vi "Dashboard Main.vi"() -> ()   [LabVIEW 2016]
uses:
  <vilib>/Utility/miscctls.llb/LVRowAndColumnTypeDef.ctl
  <vilib>/event_ctls.llb/eventvkey.ctl
  <vilib>/Rock Robotics/Network Tables/NT Read Numeric Array.vi
  <vilib>/Rock Robotics/WPI/Dashboard/WPI_DashboardLogging Global.vi
  <vilib>/Instr/_visa.llb/VISA Configure Serial Port (Instr).vi
panel:
  in  "Camera Settings Right":T1={"Frame Rate"=30, "Compression"=30, "Size"=1, "DB Camera Config"=FALSE} {"Frame Rate" scale=1.0..30.0; "Compression" scale=100.0..-1.0; "Size" items=["640x480", "320x240", "160x120"]}
  in  "Camera Name Right":string(combo)="No Camera Selection"
  out "Camera Info":cluster{"Mbps LED":bool, "Mbps":dbl, "fps":dbl} {"fps" format="%#.1g"; "Mbps" format="%#.1g"}
  in  "Camera Settings":T1={"Frame Rate"=30, "Compression"=30, "Size"=1, "DB Camera Config"=FALSE} {"Frame Rate" scale=1.0..30.0; "Compression" scale=100.0..-1.0; "Size" items=["640x480", "320x240", "160x120"]}
  in  "TCP":refnum<k5>
  in  "Rec Mode":enum32{"Stop", "Record", "Playback"}(radio)
  out "Robot IP":string
  out "Image Message":string="Timeout in Camera Communications"
  in  "Dashboard Tab":T2(tab)
  out "Boutton":bool
  out "Led2 prevstate":bool
  in  "Led2":bool
  out "Led1 prevstate":bool
  in  "Led1":bool
  in  "Select Auto":string(combo)="Select Autonomous ..."
  out "NT Connection":bool
  out "MotorChart R":cluster{"Numeric":dbl, "Numeric":dbl}(graph)
  out "MotorChart L":cluster{"Numeric":dbl, "Numeric":dbl}(graph)
  out "MotorSliders R":cluster{"MotorSlide1":dbl, "MotorSlide2":dbl} {"MotorSlide2" scale=-1.0..1.0 scale format="%#_2e"; "MotorSlide1" scale=-1.0..1.0 scale format="%#_2e"}
  out "MotorSliders L":cluster{"MotorSlide1":dbl, "MotorSlide2":dbl} {"MotorSlide2" scale=-1.0..1.0 scale format="%#_2e"; "MotorSlide1" scale=-1.0..1.0 scale format="%#_2e"}
  out "Gyro":dbl(knob) scale=0.0..360.0
  out "JS1 Z":dbl(slide) scale=-1.0..1.0 scale format="%#_2e"
  out "JS1 Graph":cluster{"X":dbl, "Y":dbl}[](graph)
  out "JS1 Buttons":T3
  out "JS2 Z":dbl(slide) scale=-1.0..1.0 scale format="%#_2e"
  out "JS2 Graph":cluster{"X":dbl, "Y":dbl}[](graph)
  out "JS2 Buttons":T3
  out "Mode":T4(ring)=enum."Auto Disabled"
  out "Camera Image Right":T5(plugin-control)
  in  "DB/String 9":string
  in  "DB/String 8":string
  in  "DB/String 7":string
  in  "DB/String 6":string
  in  "DB/String 5":string
  in  "DB/String 4":string
  in  "DB/String 3":string
  in  "DB/String 2":string
  in  "DB/String 1":string
  in  "DB/String 0":string
  in  "DB/Slider 0":dbl(slide) scale=0.0..5.0
  in  "DB/Slider 1":dbl(slide) scale=0.0..5.0
  in  "DB/Slider 2":dbl(slide) scale=0.0..5.0
  in  "DB/Slider 3":dbl(slide) scale=0.0..5.0
  out "DB/LED 3":bool
  out "DB/LED 2":bool
  out "DB/LED 1":bool
  out "DB/LED 0":bool
  in  "DB/Button 3":bool
  in  "DB/Button 2":bool
  in  "DB/Button 1":bool
  in  "DB/Button 0":bool caption="New Name"
  in  "Test Slider":dbl(slide) scale=0.0..100.0 scale format="%#_3g"
  in  "On/Off":bool caption="Solenoid"
  in  "Test Name":u16(ring) items=["Select the test to run..."]
  in  "Test Tree":string(tree)
  in  "Motor":cluster{"Value":dbl, "Enable":bool} {"Value" scale=-1.0..1.0 scale format="%#_3g"}
  out "Progress":T6 {"Test Progress" scale=0.0..100.0}
  in  "Rev/Fwd":cluster{"Forward":bool, "Reverse":bool}
  in  "Test Ring":u16(ring) items=["Monochrome", "Color"]
  out "Cmd Status":string
  in  "Execute Command":bool
  in  "Command Params":string[][](table)
  in  "Command Selection":i32(listbox)
  in  "CheckList":i32(listbox)
  out "Tree":string(tree)
  out "Camera Image":T5(plugin-control)
  out "Background":bool
  in  "Camera Name":string(combo)="No Camera Selection"
  # "HW"
  # "HW"
  # "Joysticks"
  # "Drive Motors"
  # "Front"
  # "Right"
  # "Left"
  # "Back"
  # "This tab is a great place for autonomous settings and robot-specific values.\nPlace controls and indicators inside this tab and match name to\nDashboard Variables on robot. You can also delete this comment."
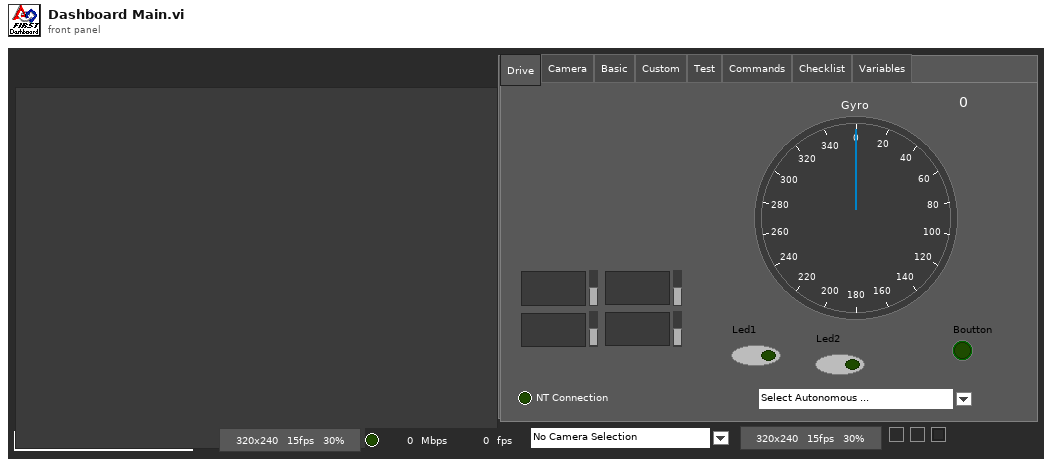
[diagram p1: front panel]
types:
  T1 = cluster{"Frame Rate":i32, "Compression":i32, "Size":u16, "DB Camera Config":bool}
  T2 = enum32{"Drive", "Camera", "Basic", "Custom", "Test", "Commands", "Checklist", "Variables"}
  T3 = cluster{bool, bool, bool, bool, bool, bool, bool, bool, bool, bool, bool, bool}
  T4 = enum8{"Tele-Op Disabled", "Tele-Op Enabled", "Auto Disabled", "Auto Enabled", "Test Disabled", "Test Enabled", "Disconnected", "No Code", "E-Stop"}
  T5 = typedef "IMAQ Image.ctl" = refnum<image>
  T6 = cluster{"Test Progress":u8, "Test Progress Text":string}
  T7 = typedef "Image Type" = u32
  T8 = cluster{"IDs":cluster{"RPC field ID":u16, "Unique ID":u16}, "String":string}
  T9 = enum32{"Drive", "Basic", "Custom", "Test", "Checklist", "Variables"}
  T10 = cluster{"Camera Image":refnum<vi>, "Dashboard Tab":refnum<vi>, "Background":refnum<vi>, "Rec Mode":refnum<vi>, "Test Slider":refnum<vi>, "On/Off ":refnum<vi>, "Test Ring":refnum<vi>, "Rev/Fwd":refnum<vi>, "Test Name":refnum<vi>, "Motor":refnum<vi>, "Progress":refnum<vi>, "CheckList":refnum<vi>, "Tree":refnum<vi>, "Test Tree":refnum<vi>, "Command Params":refnum<vi>, "Command Selection":refnum<vi>, "Execute Command":refnum<vi>, "Cmd Status":refnum<vi>, "Camera Settings":refnum<vi>, "Camera Name":refnum<vi>, "Camera Info":refnum<vi>, "Camera Settings Right":refnum<vi>, "Camera Name Right":refnum<vi>, "Camera Image Right":refnum<vi>}
  T11 = cluster{"Operation":enum16{"Update", "Clear"}, "Color Box":u32}[]
  T12 = typedef "eventvkey.ctl" = enum16{"ASCII", "Enter", "Return", "Shift", "Ctrl", "Alt", "Cmd", "Opt", "Caps", "NumLock", "Clear", "Break", "Up", "Down", "Left", "Right", "Insert", "Delete", "Home", "End", "PageUp", "PageDown", "Escape", "Help", "Pause", "ScrollLock", "F1", "F2", "F3", "F4", "F5", "F6", "F7", "F8", "F9", "F10", "F11", "F12", "F13", "F14", "F15", "F16", "F17", "F18", "F19", "F20", "F21", "F22", "F23", "F24", "Play", "VolumeUp", "VolumeDown", "Mute", "Two Byte Char"}
  T13 = cluster{"Image Size":bool, "Image Type":bool, "Pixel Value":bool, "ROI Information":bool, "Zoom Factor":bool}
  T14 = cluster{"Operation":enum16{"Update", "Clear"}, "Color Box":u32}
  T15 = typedef "LVRowAndColumnTypeDef.ctl" = cluster{"Row":i32, "Column":i32}
  T16 = cluster{"Shift":bool, "Ctrl":bool, "Alt":bool, "Cmd":bool, "Opt":bool}
  T17 = cluster{"Error Strings":string, "Disable Counts":cluster{u16, u16}, "Rail Faults":cluster{u16, u16, u16}, "Robot IP":string, "DB Mode":u8, "Event Info":cluster{"Name":string, "Type":u8, "Number":u16, "Replay":u8}}
  T18 = cluster{"Storage":cluster{"Disk Free":u64, "RAM Block":u32, "RAM free":u32}, "CPU Utilization":cluster{"CPU % ISR":sgl, "CPU % Time Crit":sgl, "CPU % Timed Str":sgl, "CPU % High":sgl, "CPU % Above":sgl, "CPU % Normal":sgl, "CPU % Low":sgl}, "CAN":cluster{"% Bus Utilization":sgl, "Bus Off Cnt":u32, "TX_FIFO Full Cnt":u32, "Receive Error Cnt":u8, "Transmit Error Cnt":u8}, "HID":cluster{"HID Outputs":u32, "Rumble Low":u16, "Rumble High":u16}[]}
  T19 = cluster{"Status bits":cluster{"Test Mode":bool, "Autonomous":bool, "Enabled":bool, "Code Start":bool, "Brownout":bool, "Reserved 2":bool, "Reserved 3":bool, "E-Stop":bool}, "Code Trace":cluster{"Disabled":bool, "TeleOp":bool, "Auto":bool, "Test":bool}, "Controller Type":enum16{"unknown", "cRIO", "roboRio"}, "Code?":enum16{"unknown", "noCode", "code"}, "Battery V":dbl}
  T20 = cluster{"Control Bits":cluster{"TestMode":bool, "Autonomous":bool, "Enabled":bool, "FMS Present":bool, bool, bool, bool, "E-Stop":bool}, "Team Station ":u8, "Countdown":sgl, "Joystick Values":cluster{"Axes":dbl[], "Buttons":bool[], "POVs":i16[]}[]}
  T21 = cluster{"Axes":dbl[], "Buttons":bool[], "POVs":i16[]}[]
  T22 = cluster{"Axes":dbl[], "Buttons":bool[], "POVs":i16[]}
  T23 = cluster{"Buttons[0]":bool, "Buttons[1]":bool, "Buttons[2]":bool, "Buttons[3]":bool, "Buttons[4]":bool, "Buttons[5]":bool, "Buttons[6]":bool, "Buttons[7]":bool, "Buttons[8]":bool, "Buttons[9]":bool, "Buttons[10]":bool, "Buttons[11]":bool}
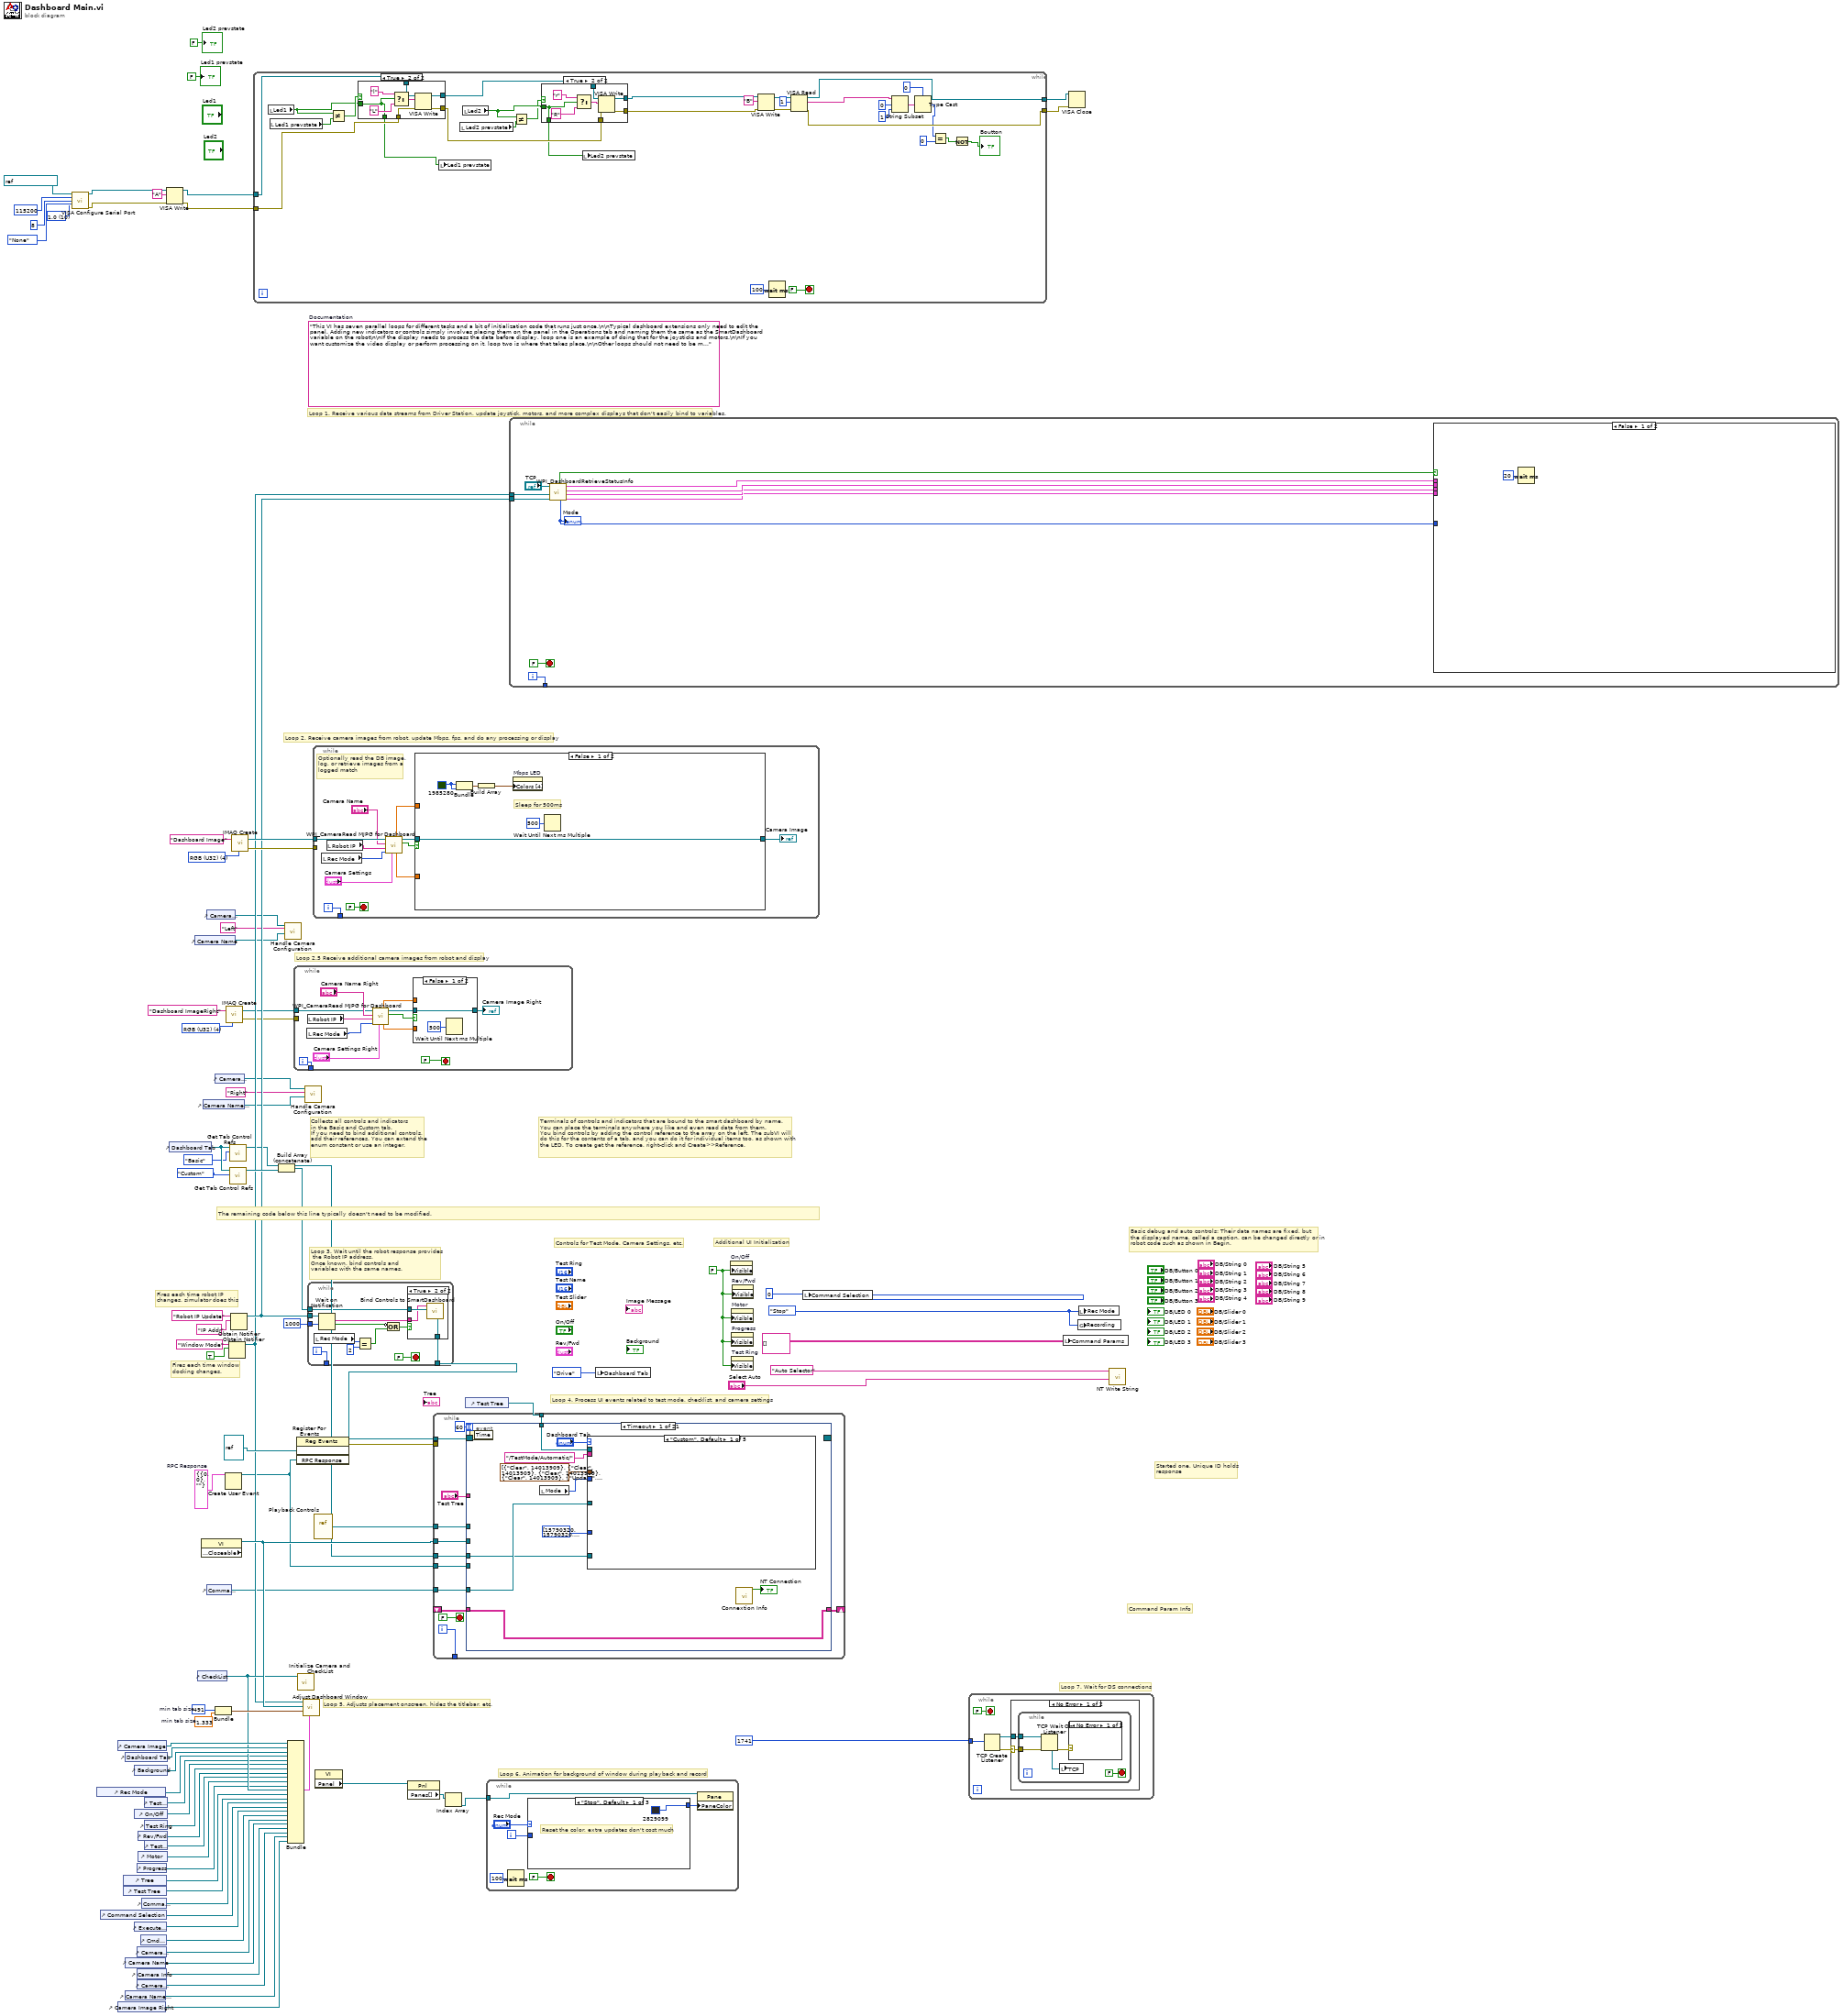
[diagram p0: block diagram]
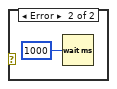
[diagram p5: hidden frame]
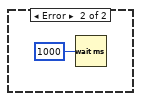
[diagram p6: hidden frame]
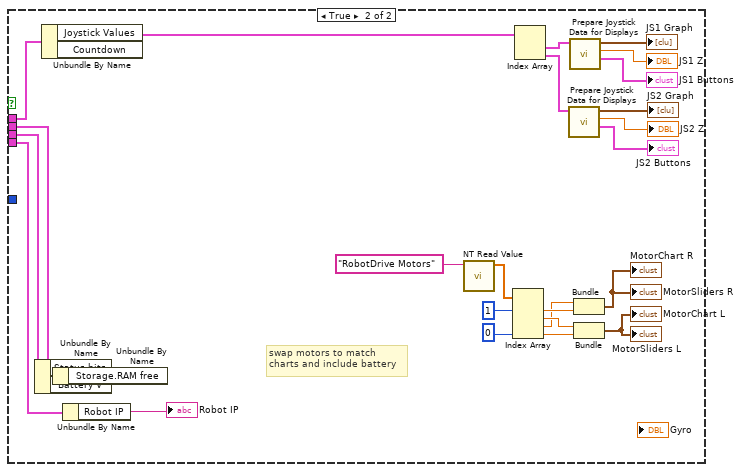
[diagram p7: hidden frame]
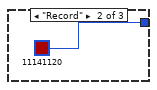
[diagram p8: hidden frame]
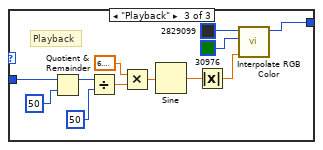
[diagram p9: hidden frame]
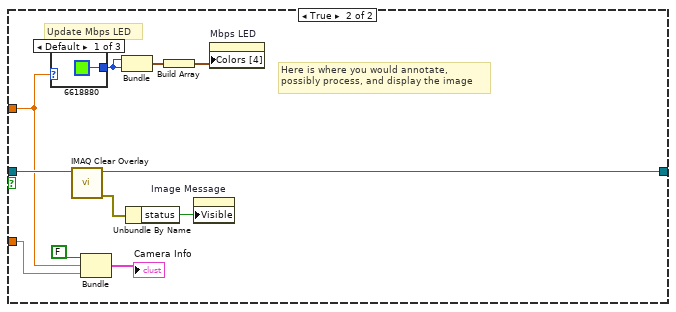
[diagram p11: hidden frame]
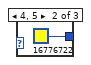
[diagram p12: hidden frame]
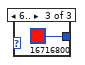
[diagram p13: hidden frame]
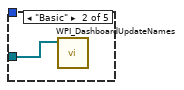
[diagram p14: hidden frame]
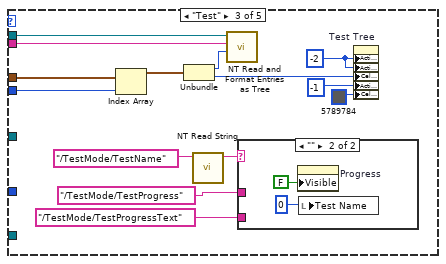
[diagram p15: hidden frame]
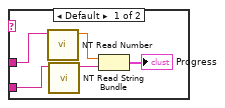
[diagram p16: hidden frame]
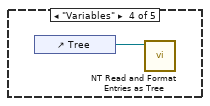
[diagram p17: hidden frame]
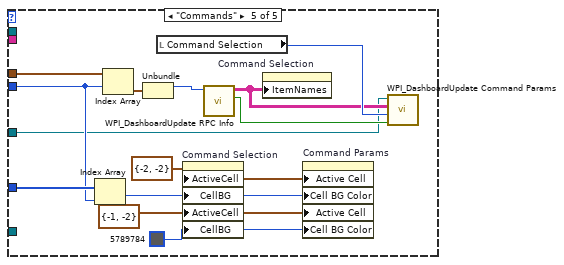
[diagram p18: hidden frame]
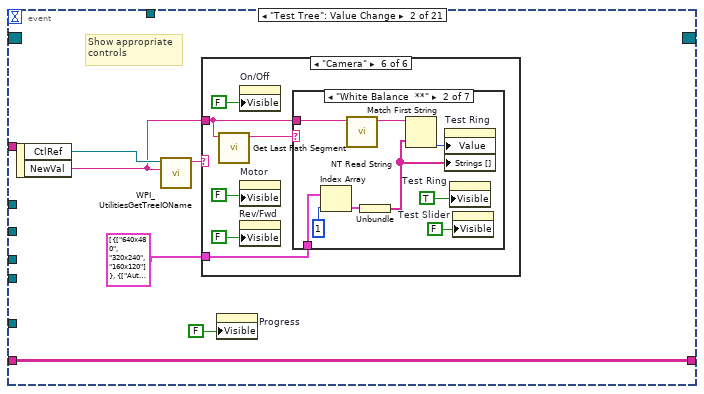
[diagram p19: hidden frame]
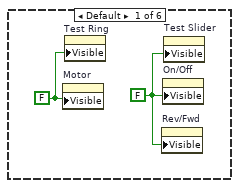
[diagram p20: hidden frame]
diagram:
  w13 = u16 10 items=["1.0"=10, "1.5"=15, "2.0"=20] ("stop bits (10: 1 bit)")
  w24 = T7 4 items=["Grayscale (U8)", "Grayscale (I16)", "Grayscale (SGL)", "Complex (CSG)", "RGB (U32)", "HSL (U32)", "RGB (U64)"] ("Image Type")
  w40 = T8 {"IDs"={"RPC field ID"=0, "Unique ID"=0}, "String"=""}  # RPC Response
  w65 = 491  # min tab size
  w64 = 1.333  # min tab size
  w72 = enum32{"Stop", "Record", "Playback"}."Stop" ("Rec Mode")
  w47 = FALSE ("Visible")
  (unwired) "This VI has seven parallel loops for different tasks and a bit of initialization code that runs just once.\n\nTypical dashboard extensions only need to edit the panel. Adding new indicators or controls simply involves placing them on the panel in the Operations tab and naming them the same as the SmartDashboard variable on the robot\n\nIf the display needs to process the data before display, loop one is an example of doing that for the joysticks and motors.\n\nIf you want customize the video display or perform processing on it, loop two is where that takes place.\n\nOther loops should not need to be modified. They are pretty standard, and document the task they perform."  # Documentation
  w89 = T7 4 items=["Grayscale (U8)", "Grayscale (I16)", "Grayscale (SGL)", "Complex (CSG)", "RGB (U32)", "HSL (U32)", "RGB (U64)"] ("Image Type")
  # "Loop 2.5 Receive additional camera images from robot and display"
  # "Command Param Info"
  # "Started one, Unique ID holds\nresponse"
  # "Loop 7. Wait for DS connections"
  # "Basic debug and auto controls: Their data names are fixed, but\nthe displayed name, called a caption, can be changed directly or in\nrobot code such as shown in Begin."
  # "Controls for Test Mode, Camera Settings, etc."
  # "Additional UI Initialization"
  # "Loop 6. Animation for background of window during playback and record"
  # "Fires each time robot IP\nchanges, simulator does this"
  # "Fires each time window\ndocking changes."
  # "Collects all controls and indicators\nin the Basic and Custom tab.\nIf you need to bind additional controls,\nadd their references. You can extend the\nenum constant or use an integer."
  # "The remaining code below this line typically doesn't need to be modified."
  # "Loop 4. Process UI events related to test mode, checklist, and camera settings"
  # "Terminals of controls and indicators that are bound to the smart dashboard by name.\nYou can place the terminals anywhere you like and even read data from them.\nYou bind controls by adding the control reference to the array on the left. The subVI will\ndo this for the contents of a tab, and you can do it for individual items too, as shown with\nthe LED. To create get the reference, right-click and Create>>Reference."
  # "Loop 3. Wait until the robot response provides\n the Robot IP address.\nOnce known, bind controls and\nvariables with the same names."
  # "Loop 5. Adjusts placement onscreen, hides the titlebar, etc."
  # "Loop 1. Receive various data streams from Driver Station, update joystick, motors, and more complex displays that don't easily bind to variables."
  # "Loop 2. Receive camera images from robot, update Mbps, fps, and do any processing or display"
  n1 = call-poly "VISA Configure Serial Port"("VISA resource name"=refnum<visa-resource-name> "ASRL4::INSTR", "baud rate (9600)"=u32 115200, "data bits (8)"=u16 8, "parity (0:none)"=enum16{"None", "Odd", "Even", "Mark", "Space"}."None", "stop bits (10: 1 bit)"=w13) -> ("VISA resource name out"=w4:refnum<visa-resource-name>, "error out"=w3:errorcluster)  [unwired: 9 in]
  n2 = control-ref of="Rec Mode"() -> (w53:refnum<vi>)
  n3 = control-ref of="Command Selection"() -> (w39:refnum<vi>)
  n4 = control-ref of="Camera Image Right"() -> (w15:refnum<vi>)
  n5 = control-ref of="Camera Image"() -> (w67:refnum<vi>)
  n6 = control-ref of="Tree"() -> (w57:refnum<vi>)
  n7 = control-ref of="Test Tree"() -> (w56:refnum<vi>)
  n8 = control-ref of="Dashboard Tab"() -> (w66:refnum<vi>)
  n9 = control-ref of="Camera Name"() -> (w30:refnum<vi>)
  n10 = control-ref of="Camera Name Right"() -> (w16:refnum<vi>)
  n11 = control-ref of="Execute Command"() -> (w41:refnum<vi>)
  n12 = control-ref of="Background"() -> (w62:refnum<vi>)
  n13 = control-ref of="On/Off"() -> (w51:refnum<vi>)
  n14 = control-ref of="Progress"() -> (w48:refnum<vi>)
  n15 = control-ref of="Camera Settings"() -> (w31:refnum<vi>)
  n16 = control-ref of="Camera Info"() -> (w29:refnum<vi>)
  n17 = control-ref of="Camera Settings Right"() -> (w17:refnum<vi>)
  n18 = control-ref of="Rev/Fwd"() -> (w49:refnum<vi>)
  n19 = control-ref of="Motor"() -> (w54:refnum<vi>)
  n20 = control-ref of="Cmd Status"() -> (w35:refnum<vi>)
  n21 = control-ref of="Command Params"() -> (w42:refnum<vi>)
  n22 = control-ref of="Test Slider"() -> (w52:refnum<vi>)
  n23 = control-ref of="Test Ring"() -> (w50:refnum<vi>)
  n24 = control-ref of="Test Name"() -> (w55:refnum<vi>)
  n25 = VISA Write(VISA resource name=w4, write buffer="A", error in (no error)=w3) -> (VISA resource name out=w6:refnum<visa-resource-name>, error out=w5:errorcluster)  [unwired: 1 out]
  n26 = control-ref of="Dashboard Tab"() -> (w70:refnum<vi>)
  n27 = control-ref of="Camera Name"() -> (w32:refnum<vi>)
  n28 = control-ref of="CheckList"() -> (w58:refnum<vi>)
  n29 = property class="VI" props=["Front Panel.Closeable"]() -> (reference out=w71:refnum<vi>)  [unwired: 2 in, 2 out]
  n30 = control-ref of="Camera Name Right"() -> (w20:refnum<vi>)
  n31 = control-ref of="Camera Settings"() -> (w33:refnum<vi>)
  n32 = control-ref of="Command Params"() -> (w34:refnum<vi>)
  n33 = control-ref of="Camera Settings Right"() -> (w21:refnum<vi>)
  n34 = Bundle("min tab size"=w65, "min tab size"=w64) -> (w63:cluster{"min tab size":i32, "min tab size":dbl})  [unwired: 1 in]
  n35 = Create User Event(user event datatype=w40) -> (user event=w36:refnum<user-event>)  [unwired: 1 in, 1 out]
  n36 = call "IMAQ Create"("Image Name"="Dashboard ImageRight", "Image Type"=w24) -> ("New Image"=w23:T5, "error out"=w22:errorcluster)  [unwired: 2 in, 1 out]
  n37 = Obtain Notifier(name (unnamed)="Window Mode", notification data type=TRUE) -> (notifier out=w45:refnum<notifier>)  [unwired: 2 in, 2 out]
  n38 = call <vilib>:"Get Tab Control Refs.vi"("Page Index"=T9."Basic" ("Dashboard Tab"), "TabControl in"=w70) -> ("ControlsOnPage"=w28:refnum<vi>[])  [unwired: 9 in]
  n39 = call <vilib>:"Get Tab Control Refs.vi"("Page Index"=T9."Custom" ("Dashboard Tab"), "TabControl in"=w70) -> ("ControlsOnPage"=w69:refnum<vi>[])  [unwired: 9 in]
  n40 = Obtain Notifier(name (unnamed)="Robot IP Update", notification data type="IP Addr" ("name (unnamed)")) -> (notifier out=w46:refnum<notifier>)  [unwired: 2 in, 2 out]
  n41 = call "IMAQ Create"("Image Name"="Dashboard Image", "Image Type"=w89) -> ("New Image"=w87:T5, "error out"=w86:errorcluster)  [unwired: 2 in, 1 out]
  n42 = while {
    tunnel: w6 -> [w115]
    tunnel: w5 -> [w114]
    tunnel: [w94] -> w7
    tunnel: [w95] -> w1
    stop <- FALSE stop-if-true
    n43 = local read "Led1"() -> (w116:bool)
    n44 = local read "Led1 prevstate"() -> (w118:bool)
    n45 = Not Equal?(x=w116, y=w118) -> (x != y?=w117:bool)
    n46 = case shown="True" w117 {
      tunnel: w116 -> [w132 w135]
      tunnel: [w133 w139] -> w110
      tunnel: [w134 w138] -> w109
      tunnel: w115 -> [w133 w137]
      tunnel: w114 -> [w134 w136]
      tunnel: [w132 w135] -> w108
      frame False {
      }
      frame True {
        n47 = Select(t="l" ("write buffer"), s=w135, f="L" ("write buffer")) -> (s? t:f=w142:string)
        n48 = VISA Write(VISA resource name=w137, write buffer=w142, error in (no error)=w136) -> (VISA resource name out=w139:refnum<visa-resource-name>, error out=w138:errorcluster)  [unwired: 1 out]
      }
    }
    n49 = local write "Led1 prevstate"(w108) -> ()
    n50 = local read "Led2 prevstate"() -> (w111:bool)
    n51 = local read "Led2"() -> (w113:bool)
    n52 = Not Equal?(x=w113, y=w111) -> (x != y?=w112:bool)
    n53 = case shown="True" w112 {
      tunnel: w113 -> [w121 w124]
      tunnel: [w122 w128] -> w106
      tunnel: [w123 w127] -> w105
      tunnel: w110 -> [w122 w126]
      tunnel: w109 -> [w123 w125]
      tunnel: [w121 w124] -> w107
      frame False {
      }
      frame True {
        n54 = Select(t="r" ("write buffer"), s=w124, f="R" ("write buffer")) -> (s? t:f=w131:string)
        n55 = VISA Write(VISA resource name=w126, write buffer=w131, error in (no error)=w125) -> (VISA resource name out=w128:refnum<visa-resource-name>, error out=w127:errorcluster)  [unwired: 1 out]
      }
    }
    n56 = local write "Led2 prevstate"(w107) -> ()
    n57 = VISA Write(VISA resource name=w106, write buffer="B", error in (no error)=w105) -> (VISA resource name out=w103:refnum<visa-resource-name>, error out=w102:errorcluster)  [unwired: 1 out]
    n58 = Wait (ms)(milliseconds to wait=u32 100) -> ()  [unwired: 1 out]
    n59 = VISA Read(VISA resource name=w103, byte count=u32 1, error in (no error)=w102) -> (VISA resource name out=w95:refnum<visa-resource-name>, read buffer=w97:string, error out=w94:errorcluster)  [unwired: 1 out]
    n60 = String Subset(string=w97, offset (0)=0, length (rest)=1 ("length (rest)")) -> (substring=w98:string)
    n61 = Type Cast(type=0 ("offset (0)"), x=w98) -> (*(type *) &x=w93:i32)
    n62 = Equal?(x=w93, y=0) -> (x = y?=w90:bool)
    n63 = Not(x=w90) -> (.not. x?=→"Boutton":bool)
  }
  n64 = Build Array (concatenate)(w28, w69) -> (w68:refnum<vi>[])
  n65 = call "Handle Camera Configuration.vi"("CameraNameRef"=w32, "Camera File Name"="Left", "ClusterRef"=w33) -> ()  [unwired: 9 in]
  n66 = Bundle("Camera Image"=w67, "Dashboard Tab"=w66, "Background"=w62, "Rec Mode"=w53, "Test Slider"=w52, "On/Off"=w51, "Test Ring"=w50, "Rev/Fwd"=w49, "Test Name"=w55, "Motor"=w54, "Progress"=w48, "CheckList"=w58, "Tree"=w57, "Test Tree"=w56, "Command Params"=w42, "Command Selection"=w39, "Execute Command"=w41, "Cmd Status"=w35, "Camera Settings"=w31, "Camera Name"=w30, "Camera Info"=w29, "Camera Settings Right"=w17, "Camera Name Right"=w16, "Camera Image Right"=w15) -> (w59:T10)  [unwired: 1 in]
  n67 = while {
    tunnel: w23 -> [w153]
    tunnel: w22 -> [_]
    tunnel: [w147] -> _
    i -> [w147]
    stop <- FALSE stop-if-true
    n68 = local read "Rec Mode"() -> (w151:enum32{"Stop", "Record", "Playback"})
    n69 = local read "Robot IP"() -> (w152:string)
    n70 = call <vilib>:"WPI_CameraRead MJPG for Dashboard.vi"("Camera Settings"="Camera Settings Right", "Rec Mode"=w151, "Robot IP"=w152, "Camera Name"="Camera Name Right", "Refnum in"=w153) -> ("Active"=w146:bool, "Refnum out"=w149:T5, "FPS"=w144:dbl, "Bandwidth (Mbps)"=w145:dbl)  [unwired: 3 in]
    n71 = case shown="False" w146 {
      tunnel: w149 -> [w155 w157]
      tunnel: w145 -> [_ _]
      tunnel: w144 -> [_ _]
      tunnel: [w155 w157] -> w143
      frame False {
        n72 = Wait Until Next ms Multiple(millisecond multiple=u32 500) -> ()  [unwired: 1 out]
      }
      frame True {
      }
    }
    "Camera Image Right" <- w143
  }
  n73 = register-events(refnum<vi> refnum, w36) -> (reference out=w76:refnum<event-registration>, error out=w75:errorcluster)  [unwired: 2 in]
  n74 = call "Initialize Camera and CheckList.vi"("ListBox in"=w58) -> ()  [unwired: 11 in]
  n75 = call "Adjust Dashboard Window.vi"("Sizing Refnums"=w59, "Size Constraints"=w63, "VI"=w71, "WIn Mode"=w45) -> ()  [unwired: 8 in]
  n76 = call "Handle Camera Configuration.vi"("CameraNameRef"=w20, "Camera File Name"="Right", "ClusterRef"=w21) -> ()  [unwired: 9 in]
  n77 = while {
    tunnel: w68 -> [w169]
    tunnel: w46 -> [w167]
    tunnel: [w165] -> _
    tunnel: u32 1000 ("milliseconds to wait") -> [w164]
    tunnel: w36 -> [w158]
    i -> [w165]
    stop <- FALSE stop-if-true
    n78 = local read "Rec Mode"() -> (w160:enum32{"Stop", "Record", "Playback"})
    n79 = Wait on Notification(notifier=w167, timeout in ms (-1)=w164) -> (notification=w166:string, timed out?=w162:bool)  [unwired: 2 in, 2 out]
    n80 = Equal?(x=w160, y=u16 2 ("Rec Mode")) -> (x = y?=w161:bool)
    n81 = Compound Arithmetic op=OR(invert w162, w161) -> (w163:bool)
    n82 = case shown="True" w163 {
      tunnel: w169 -> [_ w172]
      tunnel: w166 -> [_ w171]
      tunnel: w158 -> [_ w170]
      frame False {
      }
      frame True {
        n83 = call <vilib>:"Bind Controls to SmartDashboard.vi"("RPC ref"=w170, "Bound Control Refs"=w172, "Server IP Address"=w171) -> ()  [unwired: 9 in]
      }
    }
  }
  n84 = while {
    tunnel: w87 -> [w182]
    tunnel: w86 -> [_]
    tunnel: [w183] -> _
    i -> [w183]
    stop <- FALSE stop-if-true
    # "Optionally read the DB image,\nlog, or retrieve images from a\nlogged match"
    n85 = local read "Rec Mode"() -> (w178:enum32{"Stop", "Record", "Playback"})
    n86 = local read "Robot IP"() -> (w177:string)
    n87 = call <vilib>:"WPI_CameraRead MJPG for Dashboard.vi"("Camera Settings"="Camera Settings", "Rec Mode"=w178, "Robot IP"=w177, "Camera Name"="Camera Name", "Refnum in"=w182) -> ("Active"=w180:bool, "Refnum out"=w181:T5, "FPS"=w179:dbl, "Bandwidth (Mbps)"=w176:dbl)  [unwired: 3 in]
    n88 = case shown="False" w180 {
      tunnel: w181 -> [w185 w196]
      tunnel: w176 -> [_ w193]
      tunnel: w179 -> [_ w194]
      tunnel: [w185 w190] -> w173
      frame False {
        w187 = u32 1985280 ("Color Box")
        # "Sleep for 500ms"
        n89 = Bundle("Color Box"=w187, "Color Box"=w187) -> (w188:cluster{"Color Box":u32, "Color Box":u32})  [unwired: 1 out]
        n90 = Build Array(w188) -> (w186:cluster{"Color Box":u32, "Color Box":u32}[])
        n91 = property on="Mbps LED" class="Bool (strict)"("Colors [4]"=w186) -> ()  [unwired: 2 in, 2 out]
        n92 = Wait Until Next ms Multiple(millisecond multiple=u32 500) -> ()  [unwired: 1 out]
      }
      frame True {
        # "Here is where you would annotate,\npossibly process, and display the image"
        # "Update Mbps LED"
        n93 = case shown="Default" w193 {
          tunnel: [u32 6618880 ("Color Box") u32 16776722 ("Color Box") u32 16716800 ("Color Box")] -> w197
          frame Default {
          }
          frame 4, 5 {
          }
          frame 6.. {
          }
        }
        n94 = call "IMAQ Clear Overlay"("Image"=w196) -> ("error out"=w199:errorcluster, "Image Out"=w190:T5)  [unwired: 2 in, 7 out]
        n95 = Bundle(FALSE, "Bandwidth (Mbps)"=w193, "FPS"=w194) -> (→"Camera Info":cluster{bool, "Bandwidth (Mbps)":dbl, "FPS":dbl})  [unwired: 1 in]
        n96 = Bundle("Color Box"=w197, "Color Box"=w197) -> (w198:cluster{"Color Box":u32, "Color Box":u32})  [unwired: 1 out]
        n97 = Unbundle By Name(w199) -> ("status"=w200:bool)
        n98 = Build Array(w198) -> (w195:cluster{"Color Box":u32, "Color Box":u32}[])
        n99 = property on="Image Message" class="Str"("Visible"=w200) -> ()  [unwired: 2 in, 2 out]
        n100 = property on="Mbps LED" class="Bool (strict)"("Colors [4]"=w195) -> ()  [unwired: 2 in, 2 out]
      }
    }
    "Camera Image" <- w173
  }
  n101 = vi-ref "Playback Controls.vi"() -> (w77:refnum<vi>)
  n102 = property class="VI"() -> ("Panel"=w79:refnum<vi>)  [unwired: 2 in, 2 out]
  n103 = property class="Pnl"(reference=w79) -> ("Panes[]"=w80:refnum<vi>[])  [unwired: 1 in, 2 out]
  n104 = Index Array(array=w80) -> (element=w78:refnum<vi>)  [unwired: 1 in]
  n105 = control-ref of="Test Tree"() -> (w81:refnum<vi>)
  n106 = while {
    tunnel: [w213] -> _
    tunnel: w81 -> [w212]
    tunnel: w77 -> [w211]
    tunnel: w76 -> [w210]
    tunnel: w75 -> [_]
    tunnel: w71 -> [w209]
    tunnel: w36 -> [w208]
    tunnel: w34 -> [w207]
    shift-right: [w206] -> _
    shift-left: _ -> [w205]
    tunnel: w28 -> [w204]
    i -> [w213]
    stop <- FALSE stop-if-true
    n107 = event shown="[0] Timeout" {
      selector: w210 -> [_ _ _ _ _ _ _ _ _ _ _ _ _ _ _ _ _ _ _ _ _]
      dyn-events: [_ _ _ _ _ _ _ _ _ _ _ _ _ _ _ _ w469 _ _ _ _] -> _
      timeout: u32 60 ("milliseconds to wait") -> [_ _ _ _ _ _ _ _ _ _ _ _ _ _ _ _ _ _ _ _ _]
      tunnel: w212 -> [w225 _ _ _ _ _ _ _ _ _ _ _ _ _ _ _ _ _ _ _ _]
      tunnel: "Test Tree" -> [_ _ _ _ _ _ _ _ _ _ _ w436 w444 w446 w450 w458 _ _ _ _ _]
      tunnel: w211 -> [_ _ _ _ _ _ _ _ _ _ _ _ _ _ _ _ w471 _ w489 _ _]
      tunnel: w209 -> [_ _ _ _ _ _ _ _ _ _ _ _ _ _ _ _ w467 _ _ _ _]
      tunnel: w208 -> [_ _ _ _ _ _ _ _ _ _ _ _ _ _ _ _ w463 _ _ _ _]
      tunnel: w207 -> [w220 _ _ _ _ _ w387 _ _ _ _ _ _ _ _ _ _ _ _ _ _]
      tunnel: [w219 w264 w366 w371 w380 w384 w385 w394 w404 w411 w423 w435 w442 w445 w449 w457 w462 w484 w486 w490 w501] -> w206
      tunnel: w205 -> [w219 w264 w366 w371 w380 w384 w385 _ _ w411 w423 w435 w442 w445 w449 w457 w462 w484 w486 w490 w501]
      tunnel: w204 -> [w217 _ _ _ _ _ _ _ _ _ _ _ _ _ _ _ _ _ _ _ _]
      event Timeout {
        n108 = event-data() -> ()  [unwired: 1 in, 1 out]
        n109 = local read "Mode"() -> (w222:T4)
        n110 = case shown="\"Custom\", Default" "Dashboard Tab" {
          tunnel: w225 -> [_ _ w241 _ _]
          tunnel: "/TestMode/Automatic/" ("Name Pattern") -> [_ _ w240 _ _]
          tunnel: T11 [{"Operation"=enum."Clear", "Color Box"=14013909}, {"Operation"=enum."Clear", "Color Box"=14013909}, {"Operation"=enum."Clear", "Color Box"=14013909}, {"Operation"=enum."Clear", "Color Box"=14013909}, {"Operation"=enum."Update", "Color Box"=14013909}, {"Operation"=enum."Update", "Color Box"=16777215}, {"Operation"=enum."Clear", "Color Box"=14013909}, {"Operation"=enum."Clear", "Color Box"=14013909}, {"Operation"=enum."Clear", "Color Box"=14013909}] -> [_ _ w233 _ w257]
          tunnel: w222 -> [_ _ w232 _ w256]
          tunnel: u32[] [15790320, 15790320, 15790320, 15790320, 16777215, 16777215, 15790320, 15790320, 15790320] -> [_ _ _ _ w262]
          tunnel: w220 -> [_ _ _ _ w250]
          tunnel: w217 -> [_ w227 _ _ _]
          frame "Custom", Default {
          }
          frame "Basic" {
            n111 = call <vilib>:"WPI_DashboardUpdateNames.vi"("Controls on Tab"=w227) -> ()  [unwired: 11 in]
          }
          frame "Test" {
            w239 = -2 ("Active Item:Row Number")
            n112 = Index Array(array=w233, index=w232) -> (element=w234:T14)
            n113 = Unbundle(w234) -> ("Operation"=w235:enum16{"Update", "Clear"}, "Color Box"=w236:u32)
            n114 = call <vilib>:"NT Read String.vi"("Name"="/TestMode/TestName") -> ("String"=w230:string)  [unwired: 9 in, 1 out]
            n115 = call <vilib>:"NT Read and Format Entries as Tree.vi"("Operation"=w235, "Name Pattern"=w240, "Tree Refnum"=w241) -> ()  [unwired: 7 in, 2 out]
            n116 = case shown="\"\"" w230 {
              tunnel: "/TestMode/TestProgress" ("Name") -> [w243 _]
              tunnel: "/TestMode/TestProgressText" ("Name") -> [w242 _]
              frame Default {
                n117 = call <vilib>:"NT Read Number.vi"("Name"=w243) -> ("Numeric"=w244:dbl)  [unwired: 9 in, 1 out]
                n118 = call <vilib>:"NT Read String.vi"("Name"=w242) -> ("String"=w245:string)  [unwired: 9 in, 1 out]
                n119 = Bundle("Numeric"=w244, "String"=w245) -> (→"Progress":cluster{"Numeric":dbl, "String":string})  [unwired: 1 in]
              }
              frame "" {
                n120 = property on="Progress" class="Clust (strict)"("Visible"=FALSE) -> ()  [unwired: 2 in, 2 out]
                n121 = local write "Test Name"(u16 0) -> ()
              }
            }
            n122 = property on="Test Tree" class="Tree (strict)"("Active Item Row Number"=w239, "ActiveColNum"=w239, "CellBG"=w236, "Active Item Row Number"=-1 ("Active Item:Row Number"), "CellBG"=u32 5789784 ("Color Box")) -> ()  [unwired: 2 in, 2 out]
          }
          frame "Variables" {
            n123 = control-ref of="Tree"() -> (w249:refnum<vi>)
            n124 = call <vilib>:"NT Read and Format Entries as Tree.vi"("Tree Refnum"=w249) -> ()  [unwired: 9 in, 2 out]
          }
          frame "Commands" {
            w258 = u32 5789784 ("Color Box")
            w259 = T15 {"Row"=-1, "Column"=-2} ("Active Cell:Active Cell")
            w261 = T15 {"Row"=-2, "Column"=-2} ("Active Cell:Active Cell")
            n125 = Index Array(array=w262, index=w256) -> (element=w260:u32)
            n126 = Index Array(array=w257, index=w256) -> (element=w255:T14)
            n127 = Unbundle(w255) -> ("Operation"=w254:enum16{"Update", "Clear"})  [unwired: 1 out]
            n128 = local read "Command Selection"() -> (w253:i32)
            n129 = property on="Command Selection" class="MCListbox (strict)"("ActiveCell"=w261, "CellBG"=w260, "ActiveCell"=w259, "CellBG"=w258) -> ()  [unwired: 2 in, 2 out]
            n130 = call <vilib>:"WPI_DashboardUpdate RPC Info.vi"("Operation"=w254) -> ("update"=w252:bool, "commands"=w251:string[][])  [unwired: 9 in]
            n131 = property on="Command Selection" class="MCListbox (strict)"("ItemNames"=w251) -> ()  [unwired: 2 in, 2 out]
            n132 = property on="Command Params" class="Tbl (strict)"("Active Cell"=w261, "Cell BG Color"=w260, "Active Cell"=w259, "Cell BG Color"=w258) -> ()  [unwired: 2 in, 2 out]
            n133 = call <vilib>:"WPI_DashboardUpdate Command Params.vi"("Update"=w252, "NewVal"=w253, "Commands"=w251, "Param Tbl"=w250) -> ()  [unwired: 7 in, 1 out]
          }
        }
        n134 = call <vilib>:"Connextion Info.vi"() -> ("Connected"=→"NT Connection":bool)  [unwired: 10 in, 1 out]
      }
      event "Test Tree": Value Change {
        # "Show appropriate\ncontrols"
        n135 = event-data() -> ("CtlRef"=w267:refnum<vi>, "NewVal"=w265:string)  [unwired: 1 in]
        n136 = call <vilib>:"WPI_UtilitiesGetTreeIOName.vi"("NewVal"=w265, "TreeControl in"=w267) -> ("I/O Name"=w268:string)  [unwired: 9 in]
        n137 = case shown="\"Camera\"" w268 {
          selector: w268 -> [_ w275 _ w297 w306 _]
          tunnel: w265 -> [_ _ w294 w296 _ w313]
          tunnel: cluster{string[]}[] [{["640x480", "320x240", "160x120"]}, {["Auto", "Fixed indoor", "Fixed outdoor 1", "Fixed outdoor 2", "Fixed fluorescent 1", "Fixed fluorescent 2", "Hold current"]}, {["Auto", "Flicker-free 50 Hz", "Flicker-free 60 Hz", "Hold current"]}, {["None", "Prioritize frame rate", "Prioritize image quality"]}, {["Monochrome", "Color"]}] -> [_ _ _ _ _ w312]
          frame Default {
            w270 = FALSE ("Visible")
            w269 = FALSE ("Visible")
            n138 = property on="Motor" class="Clust (strict)"("Visible"=w269) -> ()  [unwired: 2 in, 2 out]
            n139 = property on="Test Ring" class="Ring (strict)"("Visible"=w269) -> ()  [unwired: 2 in, 2 out]
            n140 = property on="Rev/Fwd" class="Clust (strict)"("Visible"=w270) -> ()  [unwired: 2 in, 2 out]
            n141 = property on="On/Off" class="Bool (strict)"("Visible"=w270) -> ()  [unwired: 2 in, 2 out]
            n142 = property on="Test Slider" class="Slide (strict)"("Visible"=w270) -> ()  [unwired: 2 in, 2 out]
          }
          frame "Analog Out", "Motor", "PWM" {
            w276 = FALSE ("Visible")
            n143 = case shown="\"Analog Out\"" w275 {
              tunnel: [1.0 ("Value") -1.0 ("Value") 0.0 ("Value")] -> w274
              tunnel: [255.0 ("Value") 1.0 ("Value") 5.0 ("Value")] -> w273
              tunnel: [128.0 ("Value") 0.0 ("Value") 0.0 ("Value")] -> w272
              tunnel: [64.0 ("Value") 0.5 ("Value") 1.0 ("Value")] -> w271
              frame "PWM" {
              }
              frame "Motor", Default {
              }
              frame "Analog Out" {
              }
            }
            n144 = property on="Motor" class="Clust (strict)"("Visible"=TRUE) -> ()  [unwired: 2 in, 2 out]
            n145 = property on="Value" class="Slide (strict)"("Value"=w272, "Scale.Minimum"=w274, "Scale.Maximum"=w273, "Scale.Increment"=w271) -> ()  [unwired: 2 in, 2 out]
            n146 = property on="On/Off" class="Bool (strict)"("Visible"=w276) -> ()  [unwired: 2 in, 2 out]
            n147 = property on="Test Slider" class="Slide (strict)"("Visible"=w276) -> ()  [unwired: 2 in, 2 out]
            n148 = property on="Test Ring" class="Ring (strict)"("Visible"=w276) -> ()  [unwired: 2 in, 2 out]
            n149 = property on="Rev/Fwd" class="Clust (strict)"("Visible"=w276) -> ()  [unwired: 2 in, 2 out]
          }
          frame "Servo" {
            w292 = FALSE ("Visible")
            n150 = call <vilib>:"NT Read Number.vi"("Name"=w294) -> ("Numeric"=w293:dbl)  [unwired: 9 in, 1 out]
            n151 = property on="Test Slider" class="Slide (strict)"("Visible"=TRUE, "Scale.Maximum"=170.0 ("Scale.Range:Maximum")) -> ()  [unwired: 2 in, 2 out]
            n152 = local write "Test Slider"(w293) -> ()
            n153 = property on="Motor" class="Clust (strict)"("Visible"=w292) -> ()  [unwired: 2 in, 2 out]
            n154 = property on="Rev/Fwd" class="Clust (strict)"("Visible"=w292) -> ()  [unwired: 2 in, 2 out]
            n155 = property on="On/Off" class="Bool (strict)"("Visible"=w292) -> ()  [unwired: 2 in, 2 out]
            n156 = property on="Test Ring" class="Ring (strict)"("Visible"=w292) -> ()  [unwired: 2 in, 2 out]
          }
          frame "Relay", "Solenoid" {
            w295 = FALSE ("Visible")
            n157 = property on="Motor" class="Clust (strict)"("Visible"=w295) -> ()  [unwired: 2 in, 2 out]
            n158 = property on="Test Slider" class="Slide (strict)"("Visible"=w295) -> ()  [unwired: 2 in, 2 out]
            n159 = Search and Replace String(input string=w296, search string="/Value  **", replace string="/Direction") -> (result string=w302:string)  [unwired: 5 in, 3 out]
            n160 = property on="Test Ring" class="Ring (strict)"("Visible"=w295) -> ()  [unwired: 2 in, 2 out]
            n161 = call <vilib>:"NT Read String.vi"("Name"=w302) -> ("String"=w300:string)  [unwired: 9 in, 1 out]
            n162 = Equal?(x="Both directions", y=w300) -> (x = y?=w298:bool)
            n163 = Not(x=w298) -> (.not. x?=w299:bool)
            n164 = property on="Rev/Fwd" class="Clust (strict)"("Visible"=w298) -> ()  [unwired: 2 in, 2 out]
            n165 = property on="On/Off" class="Bool (strict)"("Visible"=w299, "Caption.Text"=w297) -> ()  [unwired: 2 in, 2 out]
          }
          frame "Compressor", "Digital Out" {
            w305 = FALSE ("Visible")
            # "Get direction and finish"
            n166 = property on="Motor" class="Clust (strict)"("Visible"=w305) -> ()  [unwired: 2 in, 2 out]
            n167 = property on="Test Slider" class="Slide (strict)"("Visible"=w305) -> ()  [unwired: 2 in, 2 out]
            n168 = property on="Test Ring" class="Ring (strict)"("Visible"=w305) -> ()  [unwired: 2 in, 2 out]
            n169 = property on="On/Off" class="Bool (strict)"("Visible"=TRUE, "Caption.Text"=w306) -> ()  [unwired: 2 in, 2 out]
            n170 = property on="Rev/Fwd" class="Clust (strict)"("Visible"=FALSE) -> ()  [unwired: 2 in, 2 out]
          }
          frame "Camera" {
            n171 = call <vilib>:"Get Last Path Segment.vi"("String in"=w313) -> ("String out"=w314:string)  [unwired: 10 in]
            n172 = property on="On/Off" class="Bool (strict)"("Visible"=FALSE) -> ()  [unwired: 2 in, 2 out]
            n173 = property on="Motor" class="Clust (strict)"("Visible"=FALSE) -> ()  [unwired: 2 in, 2 out]
            n174 = property on="Rev/Fwd" class="Clust (strict)"("Visible"=FALSE) -> ()  [unwired: 2 in, 2 out]
            n175 = case shown="\"White Balance  **\"" w314 {
              tunnel: w313 -> [w320 w329 w338 w347 w356 _ w362]
              tunnel: w312 -> [w318 w326 w335 w344 w353 _ _]
              frame "Size  **" {
                n176 = Index Array(array=w318) -> (element=w317:cluster{string[]})  [unwired: 1 in]
                n177 = call <vilib>:"NT Read String.vi"("Name"=w320) -> ("String"=w319:string)  [unwired: 9 in, 1 out]
                n178 = Unbundle(w317) -> (w315:string[])
                n179 = Match First String(2:w315, 3:w319) -> (0:w316:i32)  [unwired: 1 out]
                n180 = property on="Test Ring" class="Ring (strict)"("Value"=w316, "Strings []"=w315) -> ()  [unwired: 2 in, 2 out]
                n181 = property on="Test Ring" class="Ring (strict)"("Visible"=TRUE) -> ()  [unwired: 2 in, 2 out]
                n182 = property on="Test Slider" class="Slide (strict)"("Visible"=FALSE) -> ()  [unwired: 2 in, 2 out]
              }
              frame "White Balance  **" {
                n183 = Index Array(array=w326, index=1) -> (element=w327:cluster{string[]})
                n184 = call <vilib>:"NT Read String.vi"("Name"=w329) -> ("String"=w328:string)  [unwired: 9 in, 1 out]
                n185 = Unbundle(w327) -> (w324:string[])
                n186 = Match First String(2:w324, 3:w328) -> (0:w323:i32)  [unwired: 1 out]
                n187 = property on="Test Ring" class="Ring (strict)"("Value"=w323, "Strings []"=w324) -> ()  [unwired: 2 in, 2 out]
                n188 = property on="Test Ring" class="Ring (strict)"("Visible"=TRUE) -> ()  [unwired: 2 in, 2 out]
                n189 = property on="Test Slider" class="Slide (strict)"("Visible"=FALSE) -> ()  [unwired: 2 in, 2 out]
              }
              frame "Exposure  **" {
                n190 = Index Array(array=w335, index=2) -> (element=w336:cluster{string[]})
                n191 = call <vilib>:"NT Read String.vi"("Name"=w338) -> ("String"=w337:string)  [unwired: 9 in, 1 out]
                n192 = Unbundle(w336) -> (w332:string[])
                n193 = Match First String(2:w332, 3:w337) -> (0:w333:i32)  [unwired: 1 out]
                n194 = property on="Test Ring" class="Ring (strict)"("Value"=w333, "Strings []"=w332) -> ()  [unwired: 2 in, 2 out]
                n195 = property on="Test Ring" class="Ring (strict)"("Visible"=TRUE) -> ()  [unwired: 2 in, 2 out]
                n196 = property on="Test Slider" class="Slide (strict)"("Visible"=FALSE) -> ()  [unwired: 2 in, 2 out]
              }
              frame "Exposure Priority  **" {
                n197 = Index Array(array=w344, index=3) -> (element=w345:cluster{string[]})
                n198 = call <vilib>:"NT Read String.vi"("Name"=w347) -> ("String"=w346:string)  [unwired: 9 in, 1 out]
                n199 = Unbundle(w345) -> (w341:string[])
                n200 = Match First String(2:w341, 3:w346) -> (0:w342:i32)  [unwired: 1 out]
                n201 = property on="Test Ring" class="Ring (strict)"("Value"=w342, "Strings []"=w341) -> ()  [unwired: 2 in, 2 out]
                n202 = property on="Test Ring" class="Ring (strict)"("Visible"=TRUE) -> ()  [unwired: 2 in, 2 out]
                n203 = property on="Test Slider" class="Slide (strict)"("Visible"=FALSE) -> ()  [unwired: 2 in, 2 out]
              }
              frame "Color Enable  **" {
                n204 = Index Array(array=w353, index=4) -> (element=w354:cluster{string[]})
                n205 = call <vilib>:"NT Read String.vi"("Name"=w356) -> ("String"=w355:string)  [unwired: 9 in, 1 out]
                n206 = Unbundle(w354) -> (w350:string[])
                n207 = Match First String(2:w350, 3:w355) -> (0:w351:i32)  [unwired: 1 out]
                n208 = property on="Test Ring" class="Ring (strict)"("Value"=w351, "Strings []"=w350) -> ()  [unwired: 2 in, 2 out]
                n209 = property on="Test Ring" class="Ring (strict)"("Visible"=TRUE) -> ()  [unwired: 2 in, 2 out]
                n210 = property on="Test Slider" class="Slide (strict)"("Visible"=FALSE) -> ()  [unwired: 2 in, 2 out]
              }
              frame Default {
                n211 = property on="Test Ring" class="Ring (strict)"("Visible"=FALSE) -> ()  [unwired: 2 in, 2 out]
                n212 = property on="Test Slider" class="Slide (strict)"("Visible"=FALSE) -> ()  [unwired: 2 in, 2 out]
              }
              frame "Brightness  **", "Color Level  **", "Compression  **", "FPS  **", "Sharpness  **" {
                n213 = call <vilib>:"NT Read Number.vi"("Name"=w362) -> ("Numeric"=w361:dbl)  [unwired: 9 in, 1 out]
                n214 = local write "Test Slider"(w361) -> ()
                n215 = property on="Test Slider" class="Slide (strict)"("Visible"=TRUE, "Scale.Maximum"=100.0 ("Scale.Range:Maximum")) -> ()  [unwired: 2 in, 2 out]
                n216 = property on="Test Ring" class="Ring (strict)"("Visible"=FALSE) -> ()  [unwired: 2 in, 2 out]
              }
            }
          }
        }
        n217 = property on="Progress" class="Clust (strict)"("Visible"=FALSE) -> ()  [unwired: 2 in, 2 out]
      }
      event "Test Name": Mouse Enter {
        # "Populate the ring with the list of tests"
        n218 = event-data() -> ()  [unwired: 1 in, 1 out]
        n219 = call <vilib>:"NT Read String Array.vi"("Name"="/TestMode/TestList") -> ("String Array"=w370:string[])  [unwired: 9 in, 1 out]
        n220 = Build Array (concatenate)("Select the test to run...", w370) -> (w369:string[])
        n221 = property on="Test Name" class="Ring (strict)"("Strings []"=w369) -> ()  [unwired: 2 in, 2 out]
      }
      event "Test Name": Value Change {
        w372 = FALSE ("Visible")
        # "Tell the robot the test name to run"
        n222 = event-data() -> ("NewVal"=w376:u16)  [unwired: 1 in]
        n223 = property on="Test Name" class="Ring (strict)"() -> ("Strings []"=w377:string[])  [unwired: 2 in, 2 out]
        n224 = local write "Progress"(T6 {"Test Progress"=0, "Test Progress Text"=""} ("Progress")) -> ()
        n225 = Index Array(array=w377, index=w376) -> (element=w375:string)
        n226 = call <vilib>:"NT Write String.vi"("String"=w375, "Name"="/TestMode/TestName") -> ()  [unwired: 9 in, 1 out]
        n227 = property on="Progress" class="Clust (strict)"("Visible"=TRUE) -> ()  [unwired: 2 in, 2 out]
        n228 = property on="Motor" class="Clust (strict)"("Visible"=w372) -> ()  [unwired: 2 in, 2 out]
        n229 = property on="Test Slider" class="Slide (strict)"("Visible"=w372) -> ()  [unwired: 2 in, 2 out]
        n230 = property on="On/Off" class="Bool (strict)"("Visible"=w372) -> ()  [unwired: 2 in, 2 out]
        n231 = property on="Rev/Fwd" class="Clust (strict)"("Visible"=w372) -> ()  [unwired: 2 in, 2 out]
        n232 = property on="Test Ring" class="Ring (strict)"("Visible"=w372) -> ()  [unwired: 2 in, 2 out]
      }
      event "Select Auto": Mouse Enter {
        # "Populate the combo box with the list of autonomous options"
        n233 = event-data() -> ()  [unwired: 1 in, 1 out]
        n234 = call <vilib>:"NT Read String Array.vi"("Name"="Auto List") -> ("String Array"=w379:string[])  [unwired: 9 in, 1 out]
        n235 = property on="Select Auto" class="CmbBox"("Strings[]"=w379) -> ()  [unwired: 2 in, 2 out]
      }
      event "Select Auto": Value Change {
        # "User modified the Auto Selection. Write to NT variable so robot knows."
        n236 = event-data() -> ("NewVal"=w382:string)  [unwired: 1 in]
        n237 = call <vilib>:"NT Write String.vi"("String"=w382, "Name"="Auto Selector") -> ()  [unwired: 9 in, 1 out]
      }
      event "Command Selection": Value Change {
        # "Get the params and show in table"
        n238 = event-data() -> ("NewVal"=w388:i32)  [unwired: 1 in]
        n239 = property on="Command Selection" class="MCListbox (strict)"() -> ("ItemNames"=w386:string[][])  [unwired: 2 in, 2 out]
        n240 = call <vilib>:"WPI_DashboardUpdate Command Params.vi"("NewVal"=w388, "Commands"=w386, "Param Tbl"=w387) -> ()  [unwired: 8 in, 1 out]
      }
      event "Execute Command": Value Change {
        # "Started one, Unique ID holds\nresponse"
        n241 = event-data() -> ()  [unwired: 1 in, 1 out]
        n242 = property on="Command Selection" class="MCListbox (strict)"() -> ("ItemNames"=w399:string[][])  [unwired: 2 in, 2 out]
        n243 = Index Array(array=w399, index (row)="Command Selection", index (col)=0) -> (element=w397:string)
        n244 = call <vilib>:"Invoke Commands.vi"("Command Params"="Command Params", "Function Name"=w397) -> ("Params"=w393:u8, "Started"=w392:bool)  [unwired: 7 in, 1 out]
        n245 = Array Subset(array="Command Params", length (row)=w393) -> (w394:string[][])  [unwired: 3 in]
        n246 = Select(t="Executing" ("Cmd Status"), s=w392, f="" ("Cmd Status")) -> (s? t:f=→"Cmd Status":string)
      }
      event "Command Selection": Double Click {
        n247 = event-data() -> ("Row"=w407:i32)  [unwired: 1 in]
        n248 = property on="Command Selection" class="MCListbox (strict)"() -> ("ItemNames"=w410:string[][])  [unwired: 2 in, 2 out]
        n249 = local read "Command Params"() -> (w406:string[][])
        n250 = Index Array(array=w410, index (row)=w407, index (col)=0) -> (element=w408:string)
        n251 = call <vilib>:"Invoke Commands.vi"("Command Params"=w406, "Function Name"=w408) -> ("Params"=w405:u8, "Started"=w400:bool)  [unwired: 7 in, 1 out]
        n252 = Array Subset(array=w406, length (row)=w405) -> (w404:string[][])  [unwired: 3 in]
        n253 = Select(t="Executing" ("Cmd Status"), s=w400, f="" ("Cmd Status")) -> (s? t:f=w401:string)
        n254 = local write "Cmd Status"(w401) -> ()
      }
      event "CheckList": Double Click {
        # "Shift clears all"
        # "Update symbols on the listbox"
        n255 = event-data() -> ("PlatMods.Shift"=w412:bool, "Row"=w414:i32)  [unwired: 1 in]
        n256 = case shown="True" w412 {
          tunnel: w414 -> [w418 _]
          tunnel: 1 -> [w417 _]
          frame False {
            n257 = property on="CheckList" class="LstBox (strict)"() -> ("Item Symbols"=w416:i32[])  [unwired: 2 in, 2 out]
            n258 = Replace Array Subset(array=w416, new element=w417, index=w418) -> (w415:i32[])
            n259 = property on="CheckList" class="LstBox (strict)"("Item Symbols"=w415) -> ()  [unwired: 2 in, 2 out]
          }
          frame True {
            w419 = 0 ("Top Row")
            n260 = property on="CheckList" class="LstBox (strict)"() -> ("Number of Rows"=w421:u32)  [unwired: 2 in, 2 out]
            n261 = Initialize Array(0, w421) -> (w420:i32[])
            n262 = property on="CheckList" class="LstBox (strict)"("Top Row"=w419, "Value"=w419, "Item Symbols"=w420) -> ()  [unwired: 2 in, 2 out]
          }
        }
      }
      event "CheckList": Key Down {
        # "Update symbols on the listbox\nLeft and right keys check and uncheck"
        n263 = event-data() -> ("VKey"=w425:T12)  [unwired: 1 in]
        n264 = case shown="\"Left\", \"Right\"" w425 {
          selector: w425 -> [w430 _]
          tunnel: eventvkey."Left" ("VKey") -> [w428 _]
          frame "Left", "Right" {
            n265 = Equal?(x=w428, y=w430) -> (x = y?=w429:bool)
            n266 = Select(t=0, s=w429, f=1) -> (s? t:f=w431:i32)
            n267 = property on="CheckList" class="LstBox (strict)"() -> ("Item Symbols"=w434:i32[])  [unwired: 2 in, 2 out]
            n268 = Replace Array Subset(array=w434, new element=w431, index="CheckList") -> (w433:i32[])
            n269 = property on="CheckList" class="LstBox (strict)"("Item Symbols"=w433) -> ()  [unwired: 2 in, 2 out]
          }
          frame Default {
          }
        }
      }
      event "Motor.Enable": Value Change {
        # "When the test mode otor enable helper is set, update that\ntree row item's value"
        n270 = event-data() -> ("NewVal"=w440:bool)  [unwired: 1 in]
        n271 = Unbundle("Motor") -> ("Value"=w439:dbl)  [unwired: 1 out]
        n272 = Select(t=w439, s=w440, f=0.0) -> (s? t:f=w437:dbl)
        n273 = call <vilib>:"NT Write Number.vi"("Numeric"=w437, "Name"=w436) -> ()  [unwired: 9 in, 1 out]
      }
      event "Test Slider": Value Change {
        # "When the test mode slider helper is set, update that\ntree row item's value"
        n274 = event-data() -> ("NewVal"=w443:dbl)  [unwired: 1 in]
        n275 = call <vilib>:"NT Write Number.vi"("Numeric"=w443, "Name"=w444) -> ()  [unwired: 9 in, 1 out]
      }
      event "On/Off": Value Change {
        # "When the test mode on/off helper value is set, update that\ntree row item's value"
        n276 = event-data() -> ("NewVal"=w448:bool)  [unwired: 1 in]
        n277 = Boolean To (0,1)(Boolean=w448) -> (0, 1=w447:i16)
        n278 = call <vilib>:"NT Write Number.vi"("Numeric"=w447, "Name"=w446) -> ()  [unwired: 9 in, 1 out]
      }
      event "Rev/Fwd": Value Change {
        # "When the test mode helper value for relays is set, update that\ntree row item's value"
        n279 = event-data() -> ("NewVal.Forward"=w456:bool, "NewVal.Reverse"=w455:bool)  [unwired: 1 in]
        n280 = Boolean To (0,1)(Boolean=w456) -> (0, 1=w452:i16)
        n281 = Boolean To (0,1)(Boolean=w455) -> (0, 1=w454:i16)
        n282 = Negate(x=w454) -> (-x=w453:i16)
        n283 = Add(x=w452, y=w453) -> (x+y=w451:i16)
        n284 = call <vilib>:"NT Write Number.vi"("Numeric"=w451, "Name"=w450) -> ()  [unwired: 9 in, 1 out]
      }
      event "Test Ring": Value Change {
        # "When a test mode helper value is selected from the ring,\nset the tree item's variable to the string value"
        n285 = event-data() -> ("NewVal"=w460:u16)  [unwired: 1 in]
        n286 = property on="Test Ring" class="Ring (strict)"() -> ("Strings []"=w461:string[])  [unwired: 2 in, 2 out]
        n287 = Index Array(array=w461, index=w460) -> (element=w459:string)
        n288 = call <vilib>:"NT Write String.vi"("String"=w459, "Name"=w458) -> ()  [unwired: 9 in, 1 out]
      }
      event "Rec Mode": Value Change {
        # "Update globals for recording mode and path to read log from.\nClear when logging and let NetworkTables set path for vision to\nuse."
        n289 = event-data() -> ("NewVal"=w472:enum32{"Stop", "Record", "Playback"})  [unwired: 1 in]
        n290 = global write "WPI_DashboardLogging Global.vi" "Logging Filename"(path "") -> ()
        n291 = global write "WPI_DashboardLogging Global.vi" "Recording"(w472) -> ()
        n292 = case shown="\"Playback\"" w472 {
          tunnel: w471 -> [_ w474 w483]
          tunnel: [_ _ w482] -> w469
          tunnel: [_ _ w481] -> _
          tunnel: w467 -> [_ _ w479]
          tunnel: cluster{i32, i32} {-250, 170} -> [_ _ w478]
          tunnel: [_ _ T13 {"Image Size"=TRUE, "Image Type"=TRUE, "Pixel Value"=TRUE, "ROI Information"=TRUE, "Zoom Factor"=FALSE} ("Image Information Shown:All Elements")] -> w465
          tunnel: [_ _ TRUE ("Zoom Factor")] -> w464
          tunnel: w463 -> [_ _ w475]
          frame Default {
          }
          frame "Stop", "Record" {
            # "Place Window too"
            n293 = invoke class="VI" method="FP.Close"(reference=w474) -> (reference out=w473:refnum<vi>)  [unwired: 2 in, 2 out]
            n294 = invoke class="VI" method="Abort VI"(reference=w473) -> ()  [unwired: 2 in, 3 out]
          }
          frame "Playback" {
            n295 = call "Open Playback Panel.vi"("Offset"=w478, "DB VI Ref"=w479, "Playback in"=w483) -> ("Playback out"=w480:refnum<vi>)  [unwired: 8 in]
            n296 = register-events(w480, w475) -> (reference out=w482:refnum<event-registration>, error out=w481:errorcluster)  [unwired: 2 in]
          }
        }
        n297 = property on="Camera Image" class="ImageControl"("Image Information Shown"=w465, "Image Information Visible"=w464) -> ()  [unwired: 2 in, 2 out]
        n298 = call <vilib>:"WPI_DashboardNT Log FieldName Cache.vi"("Operation"=enum16{"Lookup/Add", "Index", "Clear"}."Clear") -> ()  [unwired: 8 in, 3 out]
      }
      event Panel Close {
        w485 = enum32{"Stop", "Record", "Playback"}."Stop" ("Rec Mode")
        # "Playback window has been closed, abort"
        n299 = event-data() -> ()  [unwired: 1 in, 4 out]
        n300 = local write "Rec Mode"(w485) -> ()
        n301 = global write "WPI_DashboardLogging Global.vi" "Recording"(w485) -> ()
      }
      event Panel Close {
        # "Abort playback window and ourself"
        n302 = event-data() -> ()  [unwired: 1 in, 4 out]
        n303 = invoke class="VI" method="FP.Close"(reference=w489) -> (reference out=w488:refnum<vi>)  [unwired: 2 in, 2 out]
        n304 = invoke class="VI" method="Abort VI"(reference=w488) -> (error out=w487:errorcluster)  [unwired: 2 in, 2 out]
        n305 = invoke class="VI" method="Abort VI"(error in=w487) -> ()  [unwired: 2 in, 3 out]
      }
      event User Event {
        n306 = event-data() -> ("IDs"=w496:cluster{"RPC field ID":u16, "Unique ID":u16}, "String"=w495:string)  [unwired: 1 in]
        n307 = Bundle("IDs"=w496, "String"=w495) -> (w494:T8)  [unwired: 1 in]
        n308 = call <vilib>:"Retrieve RPC Response.vi"("RPC Response"=w494) -> ("Output"=w492:string[][])  [unwired: 10 in]
        n309 = Build Array (concatenate)(w490, w492) -> (w491:string[][])
        n310 = local write "Command Params"(w491) -> ()
        n311 = local write "Cmd Status"("" ("Cmd Status")) -> ()
      }
      event "Tree": Double Click {
        n312 = event-data() -> ("PlatMods"=w500:T16, "Tag"=w499:string)  [unwired: 1 in]
        n313 = Unbundle(w500) -> ("Shift"=w498:bool)  [unwired: 4 out]
        n314 = Not(x=w498) -> (.not. x?=w497:bool)
        n315 = call <vilib>:"NT Update Persistence.vi"("Persistence"=w497, "Name"=w499) -> ()  [unwired: 9 in, 1 out]
      }
    }
  }
  n316 = while {
    tunnel: w78 -> [w503]
    i -> [w506]
    stop <- FALSE stop-if-true
    n317 = Wait (ms)(milliseconds to wait=u32 100) -> ()  [unwired: 1 out]
    n318 = case shown="\"Stop\", Default" "Rec Mode" {
      tunnel: w506 -> [_ _ w521]
      tunnel: [u32 2829099 ("Base Color") u32 11141120 ("Target Color") w510] -> w502
      frame "Stop", Default {
        # "Reset the color, extra updates don't cost much"
      }
      frame "Record" {
      }
      frame "Playback" {
        # "Playback"
        n319 = Quotient & Remainder(x=w521, y=u32 50 ("milliseconds to wait")) -> (x-y*floor(x/y)=w517:u32)  [unwired: 1 out]
        n320 = Divide(x=w517, y=u32 50 ("milliseconds to wait")) -> (x/y=w514:dbl)
        n321 = Multiply(x=6.283185307179586, y=w514) -> (x*y=w519:dbl)
        n322 = Sine(x=w519) -> (sin(x)=w518:dbl)
        n323 = Absolute Value(x=w518) -> (abs(x)=w511:dbl)
        n324 = call "Interpolate RGB Color.vi"("Proportion"=w511, "Target Color"=u32 30976, "Base Color"=u32 2829099) -> ("Result Color"=w510:u32)  [unwired: 8 in]
      }
    }
    n325 = property class="Pane"(reference=w503, "PaneColor"=w502) -> ()  [unwired: 1 in, 2 out]
  }
  n326 = while {
    tunnel: [w531] -> _
    tunnel: w46 -> [w525]
    tunnel: w45 -> [w522]
    i -> [w531]
    stop <- FALSE stop-if-true
    n327 = call <vilib>:"WPI_DashboardRetrieveStatusInfo.vi"("Binding Refnum"=w525, "Window Mode Notifier"=w522, "TCP Cnx"="TCP") -> ("Power and Errors"=w526:T17, "Robot Metrics"=w529:T18, "Status Info"=w530:T19, "Control Info"=w527:T20, "Robot Mode"=w524:T4, "Process?"=w528:bool)  [unwired: 3 in]
    "Mode" <- w524
    n328 = case shown="False" w528 {
      tunnel: w530 -> [_ w557]
      tunnel: w529 -> [_ w556]
      tunnel: w527 -> [_ w555]
      tunnel: w526 -> [_ w554]
      tunnel: w524 -> [_ _]
      frame False {
        n329 = Wait (ms)(milliseconds to wait=u32 20) -> ()  [unwired: 1 out]
      }
      frame True {
        # "swap motors to match\ncharts and include battery"
        n330 = Unbundle By Name(w557) -> ()  [unwired: 2 out]
        n331 = Unbundle By Name(w555) -> ("Joystick Values"=w545:T21)  [unwired: 1 out]
        n332 = Unbundle By Name(w556) -> ()  [unwired: 1 out]
        n333 = Unbundle By Name(w554) -> ("Robot IP"=→"Robot IP":string)
        n334 = call-poly <vilib>:"NT Read Value.vi"("Name"="RobotDrive Motors") -> ("Numeric Array"=w535:dbl[])  [unwired: 9 in, 1 out]
        n335 = Index Array(array=w535, index #1=1, index #4=0) -> (element #1=w549:dbl, element #2=w550:dbl, element #3=w548:dbl, element #4=w553:dbl)  [unwired: 2 in]
        n336 = Index Array(array=w545) -> (element #1=w544:T22, element #2=w540:T22)  [unwired: 2 in]
        n337 = call "Prepare Joystick Data for Displays.vi"("Joystick Values"=w540) -> ("Buttons"=→"JS2 Buttons":T23, "Z Axis"=→"JS2 Z":dbl, "Cartesian Data"=→"JS2 Graph":cluster{"X axis":dbl, "X axis":dbl}[])  [unwired: 8 in]
        n338 = call "Prepare Joystick Data for Displays.vi"("Joystick Values"=w544) -> ("Buttons"=→"JS1 Buttons":T23, "Z Axis"=→"JS1 Z":dbl, "Cartesian Data"=→"JS1 Graph":cluster{"X axis":dbl, "X axis":dbl}[])  [unwired: 8 in]
        n339 = Bundle("Numeric"=w548, "Numeric"=w549) -> (→"MotorChart R" →"MotorSliders R":cluster{"Numeric":dbl, "Numeric":dbl})  [unwired: 1 in]
        n340 = Bundle("Numeric"=w550, "Numeric"=w553) -> (→"MotorChart L" →"MotorSliders L":cluster{"Numeric":dbl, "Numeric":dbl})  [unwired: 1 in]
      }
    }
  }
  n341 = local write "Dashboard Tab"(T2."Drive" ("Dashboard Tab")) -> ()
  n342 = property on="On/Off" class="Bool (strict)"("Visible"=w47) -> ()  [unwired: 2 in, 2 out]
  n343 = property on="Motor" class="Clust (strict)"("Visible"=w47) -> ()  [unwired: 2 in, 2 out]
  n344 = property on="Progress" class="Clust (strict)"("Visible"=w47) -> ()  [unwired: 2 in, 2 out]
  n345 = property on="Test Ring" class="Ring (strict)"("Visible"=w47) -> ()  [unwired: 2 in, 2 out]
  n346 = property on="Rev/Fwd" class="Clust (strict)"("Visible"=w47) -> ()  [unwired: 2 in, 2 out]
  n347 = local write "Command Selection"(u16 0 ("milliseconds to wait")) -> ()
  n348 = while {
    tunnel: u16 1741 ("timeout ms (25000)") -> [w559]
    stop <- FALSE stop-if-true
    n349 = TCP Create Listener(10:w559) -> (0:w558:errorcluster, 3:w560:refnum<k5>)  [unwired: 4 in, 1 out]
    n350 = case shown="No Error" w558 {
      selector: w558 -> [w562 _]
      tunnel: w560 -> [w563 _]
      frame No Error {
        n351 = while {
          tunnel: w563 -> [w566]
          tunnel: w562 -> [w565]
          stop <- FALSE stop-if-true
          n352 = TCP Wait On Listener(8:w565, 11:w566) -> (0:w567:errorcluster, 4:w568:refnum<k5>)  [unwired: 2 in, 3 out]
          n353 = local write "TCP"(w568) -> ()
          n354 = case shown="No Error" w567 {
            frame No Error {
            }
            frame Error {
              n355 = Wait (ms)(milliseconds to wait=u32 1000) -> ()  [unwired: 1 out]
            }
          }
        }
      }
      frame Error {
        n356 = Wait (ms)(milliseconds to wait=u32 1000) -> ()  [unwired: 1 out]
      }
    }
  }
  n357 = local write "Command Params"(string[][] [] ("Command Params")) -> ()
  n358 = VISA Close(VISA resource name=w1, error in (no error)=w7) -> ()  [unwired: 1 out]
  n359 = global write "WPI_DashboardLogging Global.vi" "Recording"(w72) -> ()
  n360 = local write "Rec Mode"(w72) -> ()
  n361 = call <vilib>:"NT Write String.vi"("String"="Select Auto", "Name"="Auto Selector") -> ()  [unwired: 9 in, 1 out]
  "Led1 prevstate" <- FALSE ("Led1 prevstate")
  "Led2 prevstate" <- FALSE ("Led2 prevstate")
